vi "Initialize2.vi"(8 "error in (no error)":errorcluster, 11 "Instrument in":refnum<class "Instrument.lvclass">) -> (0 "error out":errorcluster, 3 "Instrument out":refnum<class "Instrument.lvclass">)   [LabVIEW 2012]
uses:
  Instrument.lvclass
  Comm/Stream/Stream.lvclass
  StateMachine/State Machine.lvclass
  Device/Device.lvclass
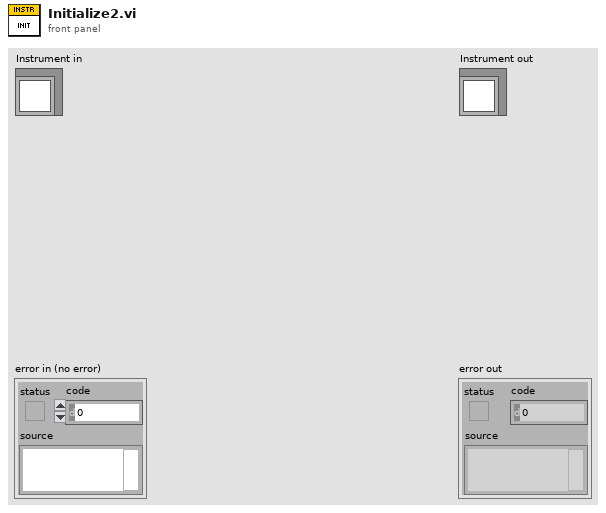
[diagram p1: front panel]
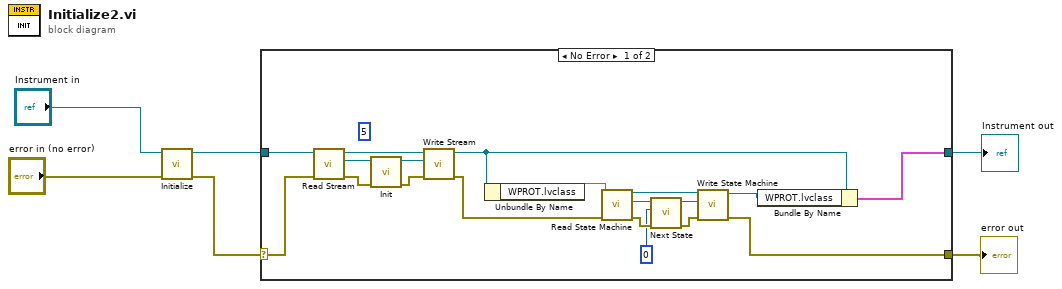
[diagram p0: block diagram]
diagram:
  n1 = call-dynamic "Initialize.vi"("error in (no error)"="error in (no error)", "Instrument in"="Instrument in") -> ("error out"=w4:errorcluster, "Instrument out"=w3:refnum<class "Instrument.lvclass">)  [unwired: 8 in]
  n2 = case shown="No Error" w4 {
    selector: w4 -> [w19 w26]
    tunnel: [w8 w27] -> w2
    tunnel: w3 -> [w25 w27]
    tunnel: [w7 w26] -> w1
    frame No Error {
      (unwired) u32 5 ("id")
      n3 = call-dynamic "Read Stream.vi"("error in (no error)"=w19, "Server in"=w25) -> ("error out"=w21:errorcluster, "Stream.lvclass"=w24:refnum<class "Stream.lvclass">, "Server out"=w23:refnum<class "Instrument.lvclass">)  [unwired: 7 in]
      n4 = call-dynamic "Init.vi"("error in (no error)"=w21, "Stream in"=w24) -> ("error out"=w20:errorcluster, "Stream out"=w22:refnum<class "Stream.lvclass">)  [unwired: 8 in]
      n5 = call-dynamic "Write Stream.vi"("error in (no error)"=w20, "Stream.lvclass"=w22, "Server in"=w23) -> ("error out"=w17:errorcluster, "Server out"=w10:refnum<class "Instrument.lvclass">)  [unwired: 7 in]
      n6 = Unbundle By Name(w10) -> ("WPROT.lvclass"=w18)
      n7 = call-dynamic "Read State Machine.vi"("error in (no error)"=w17, "Device in"=w18) -> ("error out"=w13:errorcluster, "State Machine.lvclass"=w16:refnum<class "State Machine.lvclass">, "Device out"=w15:refnum<class "Device.lvclass">)  [unwired: 7 in]
      n8 = call "Next State.vi"("error in (no error)"=w13, "New_State"=0, "State Machine in"=w16) -> ("error out"=w12:errorcluster, "State Machine out"=w14:refnum<class "State Machine.lvclass">)  [unwired: 7 in]
      n9 = call-dynamic "Write State Machine.vi"("error in (no error)"=w12, "State Machine.lvclass"=w14, "Device in"=w15) -> ("error out"=w7:errorcluster, "Device out"=w9:refnum<class "Device.lvclass">)  [unwired: 7 in]
      n10 = Bundle By Name(cluster=w10, "WPROT.lvclass"=w9) -> (w8:cluster{})
    }
    frame Error {
    }
  }
  "error out" <- w1
  "Instrument out" <- w2
